vi "Read Multiple.vi"(0 "VISA resource name":refnum<visa-resource-name>, 1 "Source (0: Function)":u16(ring) items=["Function", "Calculation 1"], 2 "Format (0: ASCII)":u16(ring) items=["ASCII", "Single Precision", "Double Precision"], 3 "Number of Readings (100)":i32=100, 4 "Sample Count (1)":i32=1, 5 "error in (no error)":errorcluster, 8 "Timeout (25000 ms)":u32=25000) -> (14 "VISA resource name out":refnum<visa-resource-name>, 15 "Data":dbl[](array[numeric]), 16 "Channels":i32[](array[numeric]), 17 "Units":string[](array[string]), 19 "error out":errorcluster)   [LabVIEW 2016, in "Keithley 2182A.lvlib"]
doc: "This VI reads multiple measurements or calculations from the instrument. This VI should be used instead of the Data Read Single VI when you plan on reading many measurements at once or when you are reading measurements from many channels."
uses:
  <instrlib>/Keithley 2182A/Keithley 2182A.lvlib
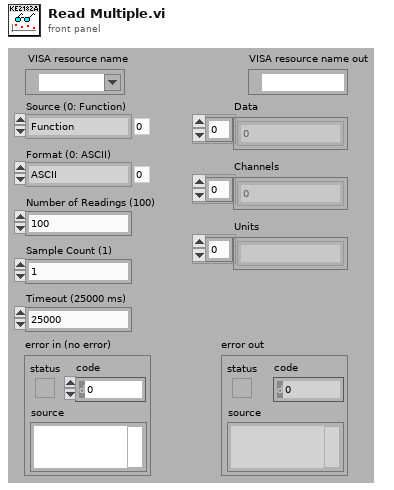
[diagram p1: front panel]
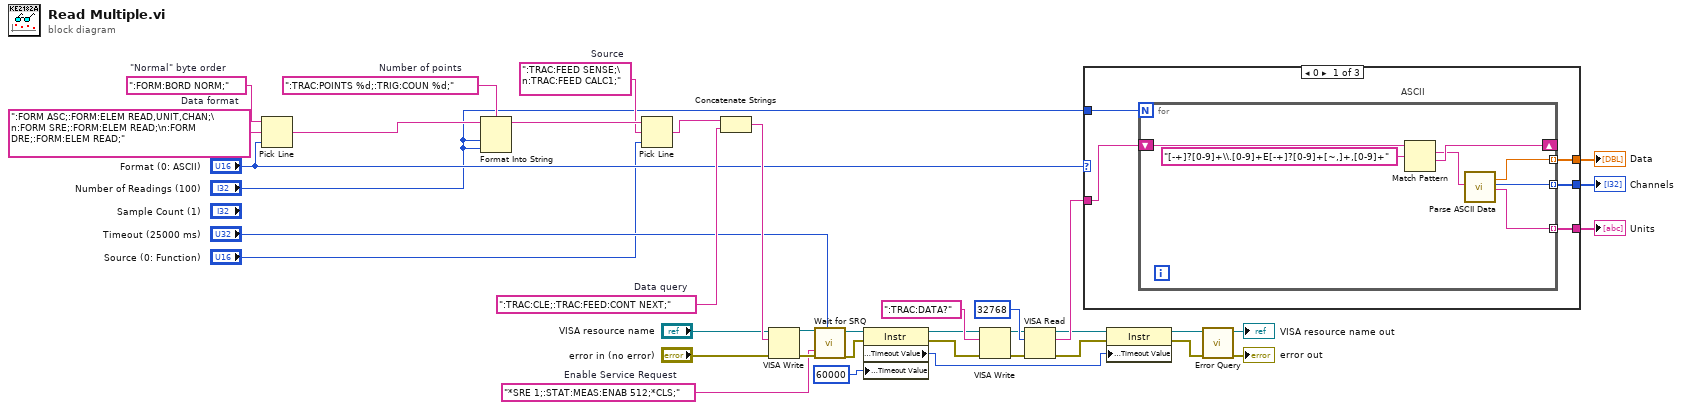
[diagram p0: block diagram]
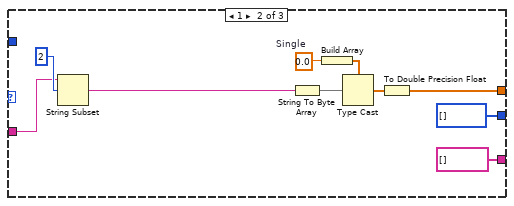
[diagram p2: hidden frame]
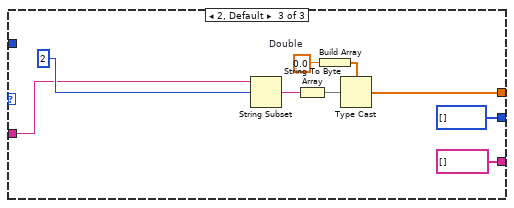
[diagram p3: hidden frame]
diagram:
  w20 = ":TRAC:FEED SENSE;\n:TRAC:FEED CALC1;"  # Source
  w2 = "*SRE 1;:STAT:MEAS:ENAB 512;*CLS;"  # Enable Service Request
  w35 = ":TRAC:POINTS %d;:TRIG:COUN %d;"  # Number of points
  w36 = ":FORM:BORD NORM;"  # "Normal" byte order
  w37 = ":FORM ASC;:FORM:ELEM READ,UNIT,CHAN;\n:FORM SRE;:FORM:ELEM READ;\n:FORM DRE;:FORM:ELEM READ;"  # Data format
  w33 = ":TRAC:CLE;:TRAC:FEED:CONT NEXT;"  # Data query
  n1 = Pick Line(string ("")=w36, multi-line string=w37, line index="Format (0: ASCII)") -> (output string=w34:string)
  n2 = Format Into String(format string=w35, initial string=w34, "Number of Readings (100)", "Number of Readings (100)") -> (resulting string=w23:string)  [unwired: 1 in, 1 out]
  n3 = Pick Line(string ("")=w23, multi-line string=w20, line index="Source (0: Function)") -> (output string=w21:string)
  n4 = Concatenate Strings(w21, w33) -> (w32:string)
  n5 = VISA Write(VISA resource name="VISA resource name", write buffer=w32, error in (no error)="error in (no error)") -> (VISA resource name out=w27:refnum<visa-resource-name>, error out=w28:errorcluster)  [unwired: 1 out]
  n6 = call <instrlib>:"Wait for SRQ.vi"("VISA resource name"=w27, "SRQ Enable Command"=w2, "error in (no error)"=w28, "Timeout (25000 ms)"="Timeout (25000 ms)") -> ("VISA resource name out"=w16:refnum<visa-resource-name>, "error out"=w15:errorcluster)  [unwired: 14 in]
  n7 = property class="Instr"(reference=w16, error in=w15, "General Settings:Timeout Value"=u32 60000) -> (reference out=w13:refnum<visa-resource-name>, error out=w12:errorcluster, "General Settings:Timeout Value"=w11:u32)
  n8 = VISA Write(VISA resource name=w13, write buffer=":TRAC:DATA?", error in (no error)=w12) -> (VISA resource name out=w18:refnum<visa-resource-name>, error out=w19:errorcluster)  [unwired: 1 out]
  n9 = VISA Read(VISA resource name=w18, byte count=u32 32768, error in (no error)=w19) -> (VISA resource name out=w10:refnum<visa-resource-name>, read buffer=w30:string, error out=w9:errorcluster)  [unwired: 1 out]
  n10 = case shown="0" "Format (0: ASCII)" {
    tunnel: [w42 w57 w63] -> w29
    tunnel: w30 -> [w43 w55 w65]
    tunnel: [w41 string[] [] string[] []] -> w25
    tunnel: [w40 i32[] [] i32[] []] -> w24
    tunnel: "Number of Readings (100)" -> [w39 _ _]
    frame 0 {
      # "ASCII"
      n11 = for {
        N: w39 -> [_]
        shift-right: [w49] -> _
        shift-left: w43 -> [w50]
        tunnel: [w46] -> w42 mode=indexing
        tunnel: [w45] -> w41 mode=indexing
        tunnel: [w44] -> w40 mode=indexing
        n12 = Match Pattern(string=w50, regular expression="[-+]?[0-9]+\\.[0-9]+E[-+]?[0-9]+[~,]+,[0-9]+") -> (match substring=w47:string, after substring=w49:string)  [unwired: 1 in, 2 out]
        n13 = call <instrlib>:"Parse ASCII Data.vi"("ASCII Data (Empty)"=w47) -> ("Measurement"=w46:dbl, "Channel"=w44:i32, "Units"=w45:string)  [unwired: 16 in]
      }
    }
    frame 1 {
      w60 = sgl 0.0  # Single
      n14 = String Subset(string=w55, offset (0)=2) -> (substring=w54:string)  [unwired: 1 in]
      n15 = String To Byte Array(string=w54) -> (unsigned byte array=w58:u8[])
      n16 = Build Array(w60) -> (w59:sgl[])
      n17 = Type Cast(type=w59, x=w58) -> (*(type *) &x=w53:sgl[])
      n18 = To Double Precision Float(number=w53) -> (double precision float=w57:dbl[])
    }
    frame 2, Default {
      w69 = 0.0  # Double
      n19 = String Subset(string=w65, offset (0)=2) -> (substring=w64:string)  [unwired: 1 in]
      n20 = String To Byte Array(string=w64) -> (unsigned byte array=w67:u8[])
      n21 = Build Array(w69) -> (w68:dbl[])
      n22 = Type Cast(type=w68, x=w67) -> (*(type *) &x=w63:dbl[])
    }
  }
  "Data" <- w29
  "Channels" <- w24
  "Units" <- w25
  n23 = property class="Instr"(reference=w10, error in=w9, "General Settings:Timeout Value"=w11) -> (reference out=w8:refnum<visa-resource-name>, error out=w7:errorcluster)
  n24 = call <instrlib>:"Error Query.vi"("error in (no error)"=w7, "VISA resource name"=w8) -> ("error out"=→"error out":errorcluster, "VISA resource name out"=→"VISA resource name out":refnum<visa-resource-name>)  [unwired: 6 in, 2 out]
